vi "Read U32.vi"(11 "unsigned byte array":u8[](array[numeric])) -> (3 "U32 Out":u32, 5 "rest of array":u8[](array[numeric]))   [LabVIEW 2015]
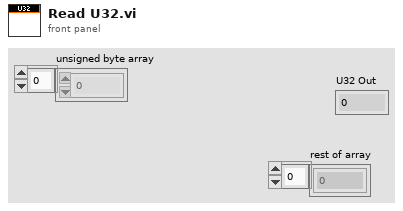
[diagram p1: front panel]
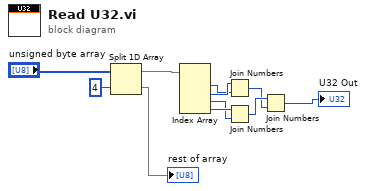
[diagram p0: block diagram]
diagram:
  n1 = Split 1D Array(array="unsigned byte array", index=4) -> (first subarray=w5:u8[], second subarray=→"rest of array":u8[])
  n2 = Index Array(array=w5) -> (element #1=w6:u8, element #2=w7:u8, element #3=w8:u8, element #4=w9:u8)  [unwired: 4 in]
  n3 = Join Numbers(hi=w7, lo=w6) -> ((hi.lo)=w10:u16)
  n4 = Join Numbers(hi=w9, lo=w8) -> ((hi.lo)=w11:u16)
  n5 = Join Numbers(hi=w11, lo=w10) -> ((hi.lo)=→"U32 Out":u32)
